vi "Read Data.vi"(7 "SlaveID":u8=1, 8 "error in (no error)":errorcluster, 9 "# samples to read":u16, 11 ".NET Refnum in":refnum<k24>) -> (0 "error out":errorcluster, 1 "# samples in buffer":u16, 2 "Vib":u16[](array[numeric]), 3 "reference out":refnum<k24>)   [LabVIEW 2017]
uses:
  C:/Users/chrisjan/Desktop/NowWorking/ITRI/DLL/Modbus.dll
  DLL/Modbus.dll
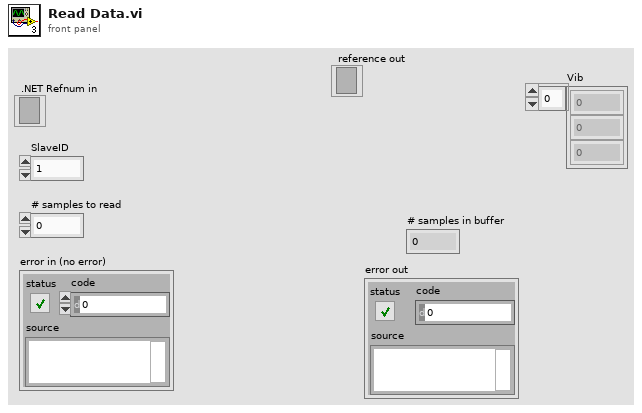
[diagram p1: front panel]
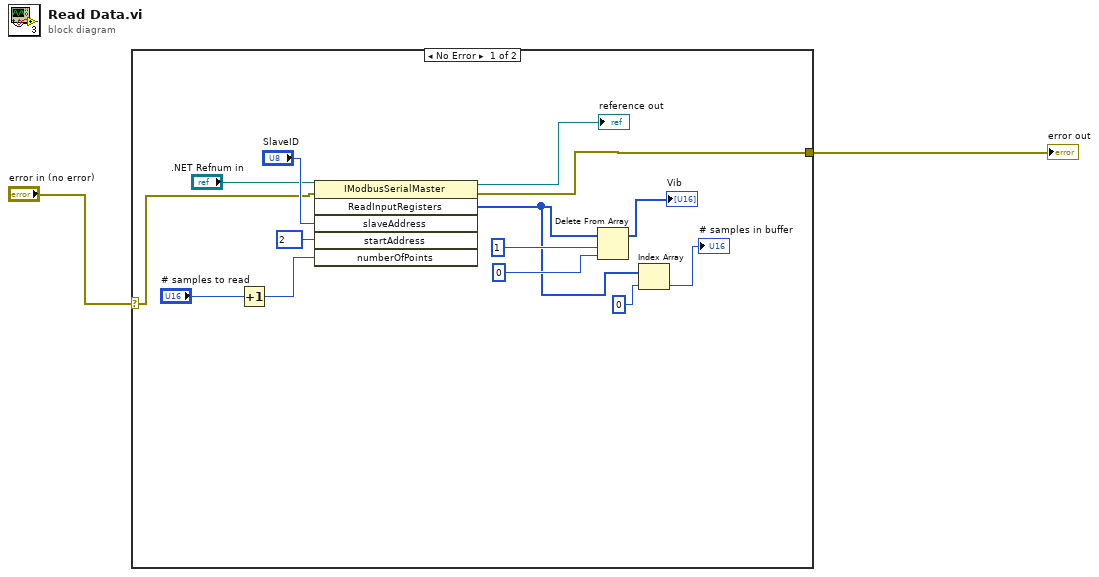
[diagram p0: block diagram]
diagram:
  n1 = case shown="No Error" "error in (no error)" {
    selector: "error in (no error)" -> [w3 w17]
    tunnel: [w8 w17] -> w2
    frame No Error {
      n2 = Increment(x="# samples to read") -> (x+1=w5:u16)
      n3 = invoke class="IModbusSerialMaster" method="ReadInputRegisters"(reference=".NET Refnum in", error in=w3, "slaveAddress"="SlaveID", "startAddress"=u16 2, "numberOfPoints"=w5) -> (reference out=→"reference out":refnum<k24>, error out=w8:errorcluster, "ReadInputRegisters"=w6:u16[])  [unwired: 1 in, 3 out]
      n4 = Delete From Array(array=w6, length=1, index=0) -> (array with subset deleted=→"Vib":u16[])  [unwired: 1 out]
      n5 = Index Array(array=w6, index=0) -> (element=→"# samples in buffer":u16)
    }
    frame Error {
    }
  }
  "error out" <- w2
